vi "SetWidthHeightToMinimum.vi"(11 "Limited Height Width in":T1) -> (3 "Limited Height Width out":T1)   [LabVIEW 2022 SP3, in "PentaPanesLibrary.lvlib" / "PentaPanes.lvclass"]
uses:
  PentaPanes.lvclass
  <vilib>/Utility/miscctls.llb/LVBoundsTypeDef.ctl
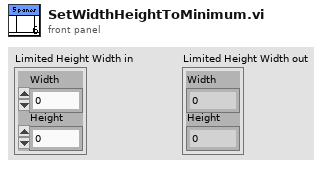
[diagram p1: front panel]
types:
  T1 = typedef "LVBoundsTypeDef.ctl" = cluster{"Width":i32, "Height":i32}
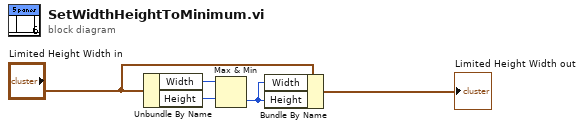
[diagram p0: block diagram]
diagram:
  n1 = Unbundle By Name("Limited Height Width in") -> ("Width"=w2:i32, "Height"=w1:i32)
  n2 = Max & Min(x=w2, y=w1) -> (min(x,y)=w3:i32)  [unwired: 1 out]
  n3 = Bundle By Name(cluster="Limited Height Width in", "Width"=w3, "Height"=w3) -> (→"Limited Height Width out":T1)
